vi "Header Footer Transform Header Footer [ ] V3.vi"(7 "Header or Footer [ ]":T15, 11 "error in (no error)":errorcluster) -> (8 "Header or Footer Complete Cluster":T1, 15 "error out":errorcluster)   [LabVIEW 2019, in "Exaprom PDF.lvlib"]
doc: "Version 1.0\nDeveloped by Jean-Marc Simard\nCopyright © 2010, Exaprom Inc.\nAll rights reserved.\nLicense: BSD\n\nWith iTextSharp 4.1.6 (http://itextsharp.sourceforge.net)\nunder Mozilla Public License Version 1.1\n(http://www.mozilla.org/MPL/MPL-1.1.html)"
uses:
  Exaprom PDF.lvlib
  LV Class/Header and Footer Class/VIs/Controls/Header Footer [ ] V2.ctl
  LV Class/Header and Footer Class/VIs/Controls/Header Footer cluster V2.ctl
  Controls/Header, Footer and Watermark Controls/Header or Footer.ctl
  Controls/Header, Footer and Watermark Controls/Header Footer Type.ctl
  Controls/Header, Footer and Watermark Controls/Header footer horiz alignment.ctl
  Controls/Table Controls/Cell Vertical alignment.ctl
  Controls/Text Controls/Line spacing.ctl
  Controls/Header, Footer and Watermark Controls/Page number.ctl
  Controls/Font Controls/Font complete cluster horizontal.ctl
  Controls/Font Controls/Font size.ctl
  Controls/Font Controls/Font color.ctl
  Controls/Font Controls/Type and encoding.ctl
  Controls/Text Controls/Unicode/Type and run direction.ctl
  C:/work/niobrara_lv/labview pdf writer fixing/DLL/itextsharp.dll
  DLL/itextsharp.dll
  Controls/Header, Footer and Watermark Controls/Header Footer Line.ctl
  Controls/Header, Footer and Watermark Controls/Header Footer Complete Cluster.ctl
  Controls/Header, Footer and Watermark Controls/Header or Footer Position.ctl
  Controls/Header, Footer and Watermark Controls/Header Footer Cluster with references.ctl
  Controls/Text Controls/Text type.ctl
  LV Class/Header and Footer Class/Header and Footer Class.lvclass
panel:
  # "X"
  # "Y"
  # "X"
  # "Y"
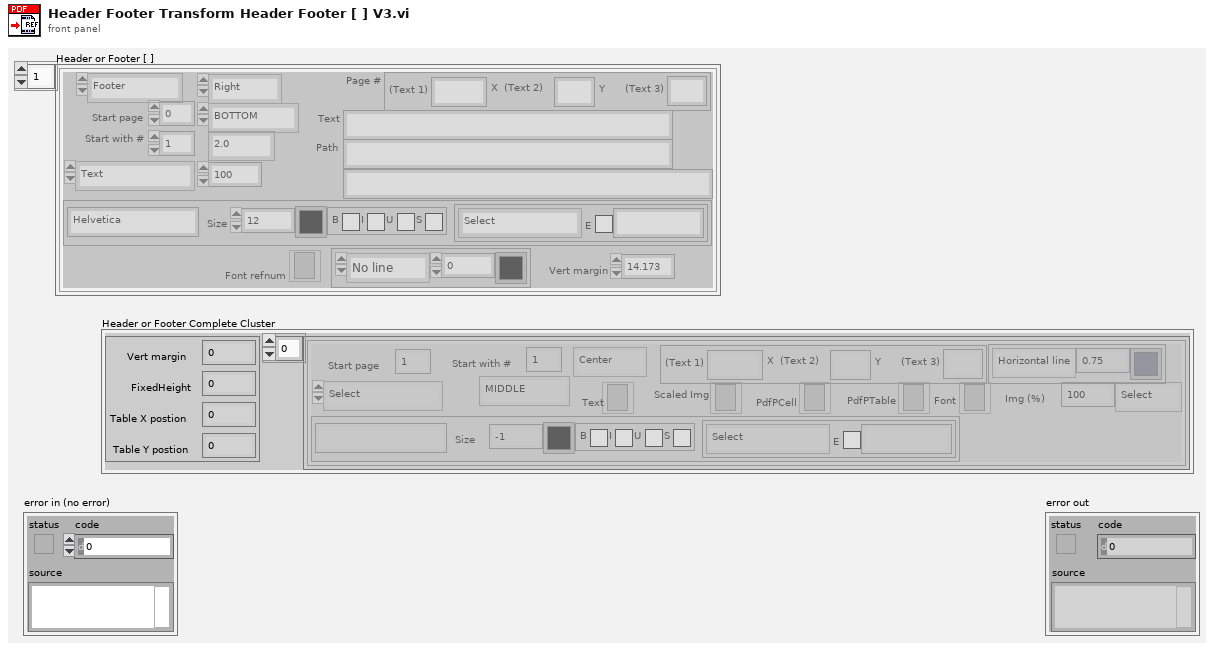
[diagram p1: front panel]
types:
  T1 = typedef "Exaprom PDF.lvlib/Header Footer Complete Cluster.ctl" = cluster{"Table position":T2, "Header Footer Cluster with references [ ]":T3[]}
  T2 = typedef "Exaprom PDF.lvlib/Header or Footer Position.ctl" = cluster{"Vert margin":dbl, "FixedHeight":dbl, "Table X postion":dbl, "Table Y postion":dbl}
  T3 = typedef "Exaprom PDF.lvlib/Header Footer Cluster with references.ctl" = cluster{"Start page":i32, "Type":T4, "Start with #":i32, "Alignment":T5, "Vertical Alignement":T6, "Page #":T7, "Text":refnum<k24>, "Scaled Img":refnum<k24>, "PdfPCell":refnum<k24>, "PdfPTable":refnum<k24>, "Font Cluster":T8, "Font ":refnum<k24>, "Img (%)":sgl, "Line":cluster{"Line":T13, "Thickness (points)":sgl, "Colour":T10}, "Line spacing":T14}
  T4 = typedef "Exaprom PDF.lvlib/Header Footer Type.ctl" = enum16{"Select", "Text", "Text + hyperlink", "Page number", "Image", "Image + hyperlink"}
  T5 = typedef "Exaprom PDF.lvlib/Header footer horiz alignment.ctl" = enum16{"Left", "Center", "Right"}
  T6 = typedef "Exaprom PDF.lvlib/Cell Vertical alignment.ctl" = enum16{"TOP", "MIDDLE", "BOTTOM"}
  T7 = typedef "Exaprom PDF.lvlib/Page number.ctl" = cluster{"Text 1":string, "Text 2":string, "Text 3":string}
  T8 = typedef "Exaprom PDF.lvlib/Font complete cluster horizontal.ctl" = cluster{"Name":string, "Size":T9, "Color":T10, "Style":cluster{"Bold":bool, "Italic":bool, "Underline":bool, "Strikeout":bool}, "Type":T11}
  T9 = typedef "Exaprom PDF.lvlib/Font size.ctl" = sgl
  T10 = typedef "Exaprom PDF.lvlib/Font color.ctl" = u32
  T11 = typedef "Exaprom PDF.lvlib/Type and encoding.ctl" = cluster{"Type&direction":T12, "Embedded":bool, "Encoding":string}
  T12 = typedef "Exaprom PDF.lvlib/Type and run direction.ctl" = enum16{"Select", "ASCII", "UTF-16", "UTF-16 (default)", "UTF-16 (LTR)", "UTF-16 (RTL)"}
  T13 = typedef "Exaprom PDF.lvlib/Header Footer Line.ctl" = enum16{"No line", "Horizontal line"}
  T14 = typedef "Exaprom PDF.lvlib/Line spacing.ctl" = enum16{"Select", "1.0", "1.5", "2.0"}
  T15 = typedef "Exaprom PDF.lvlib/Header and Footer Class.lvclass/Header Footer [ ] V2.ctl" = T16[]
  T16 = typedef "Exaprom PDF.lvlib/Header and Footer Class.lvclass/Header Footer cluster V2.ctl" = cluster{"Header or Footer":T17, "Start page":i32, "Start with #":i32, "Type":T4, "Alignment":T5, "Vertical Alignement":T6, "Line spacing":T14, "Image (%)":sgl, "Page #":T7, "Text":string, "Path":string, "Font":T8, "Font refnum":refnum<k24>, "Line":cluster{"Line":T13, "Thickness (points)":sgl, "Colour":T10}, "Vert margin":dbl, "Hyperlink":string}
  T17 = typedef "Exaprom PDF.lvlib/Header or Footer.ctl" = enum16{"Header", "Footer"}
  T18 = typedef "Exaprom PDF.lvlib/Text type.ctl" = enum16{"empty", "Text", "Hyperlink"}
  T19 = cluster{"Text type":T18, "Text":string, "Hyperlink":string}[]
  T20 = cluster{"Text type":T18, "Text":string, "Hyperlink":string}
  T21 = cluster{"Line":T13, "Thickness (points)":sgl, "Colour":T10}
  T22 = cluster{"Table position":T2, "Header Footer Cluster with references [ ]":T3[]}
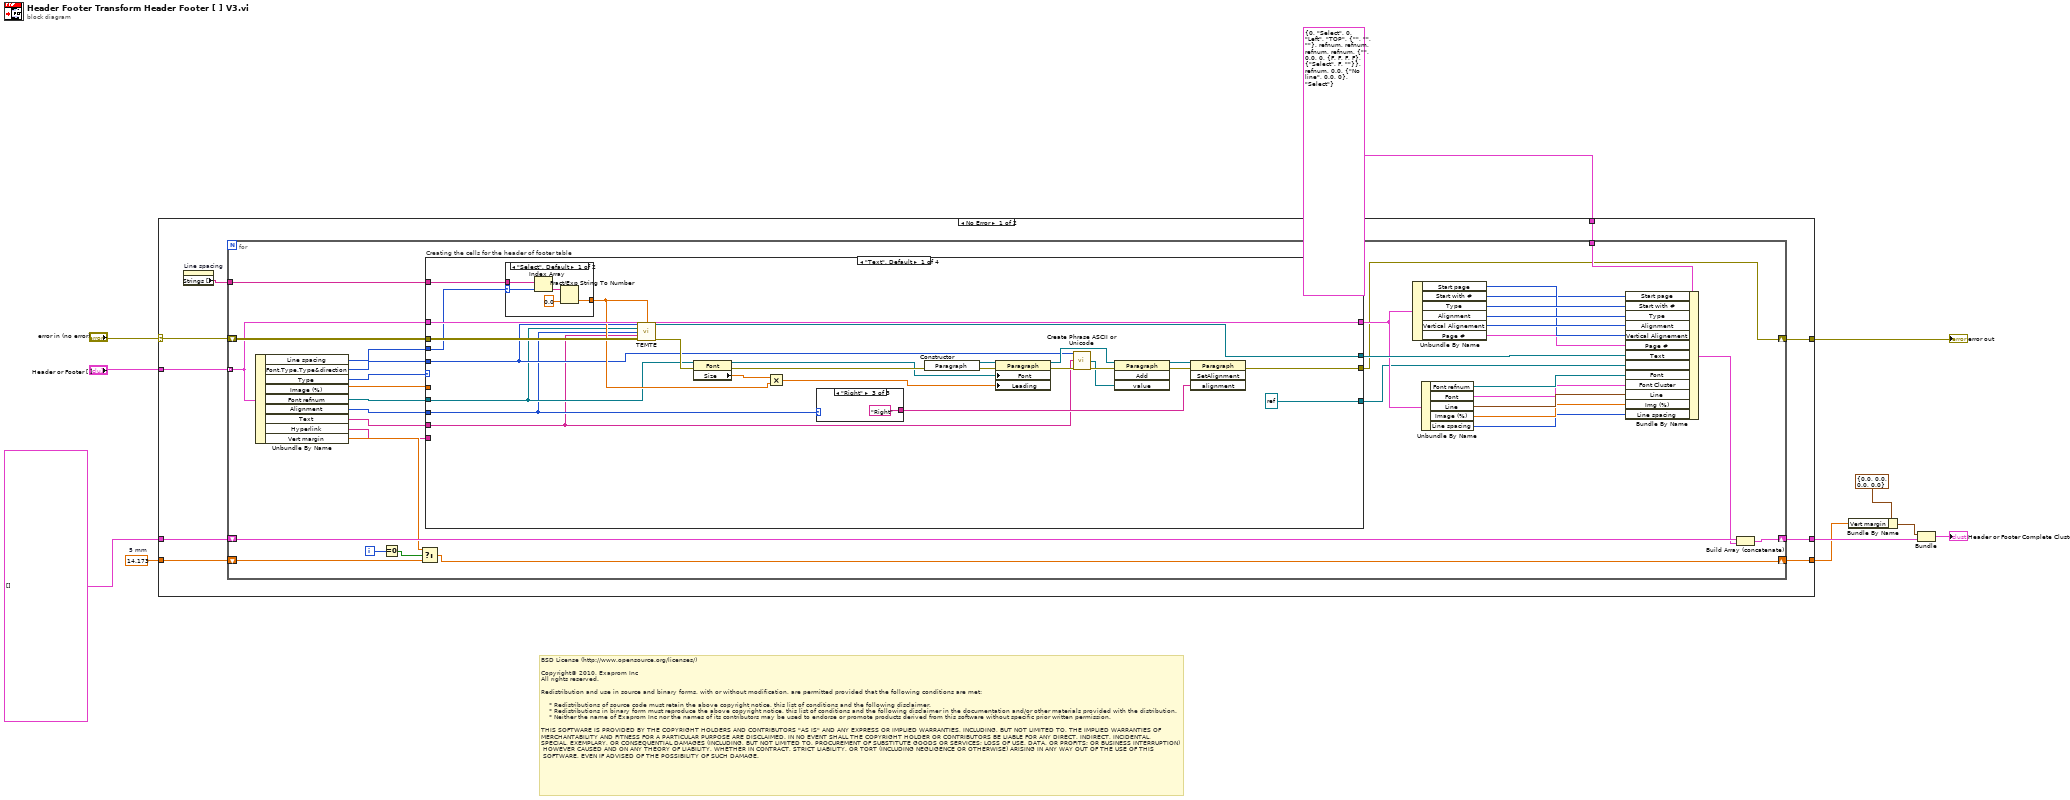
[diagram p0: block diagram]
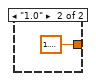
[diagram p2: hidden frame]
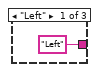
[diagram p3: hidden frame]
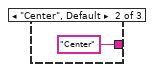
[diagram p4: hidden frame]
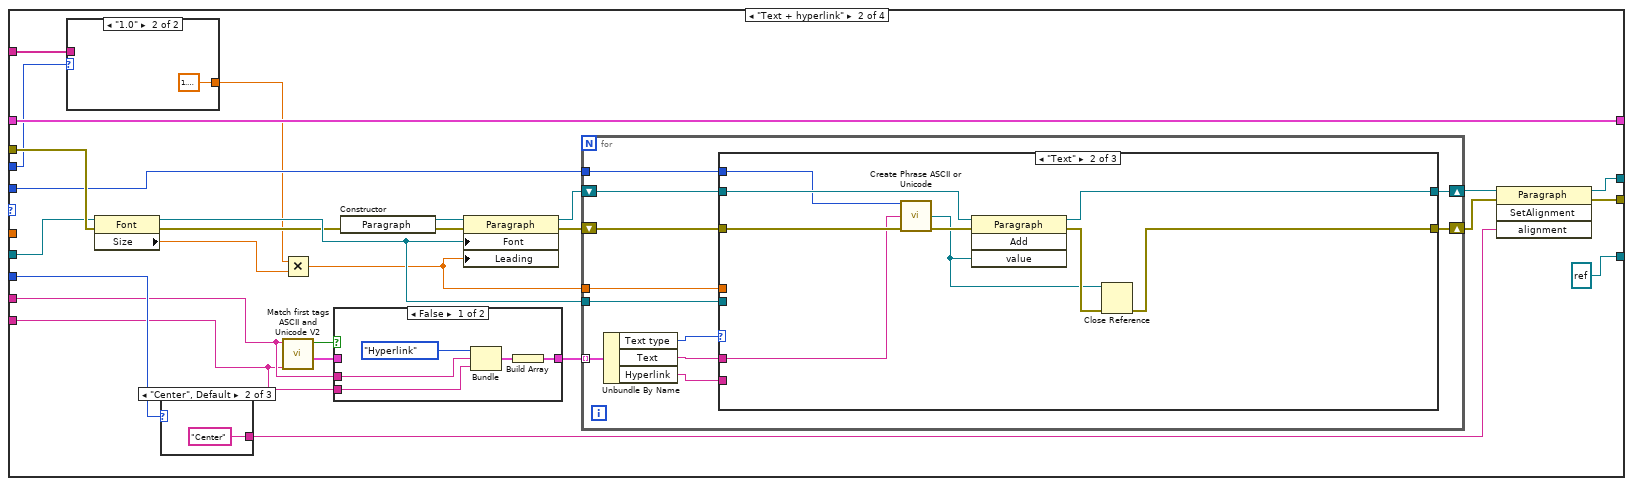
[diagram p5: hidden frame]
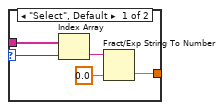
[diagram p6: hidden frame]
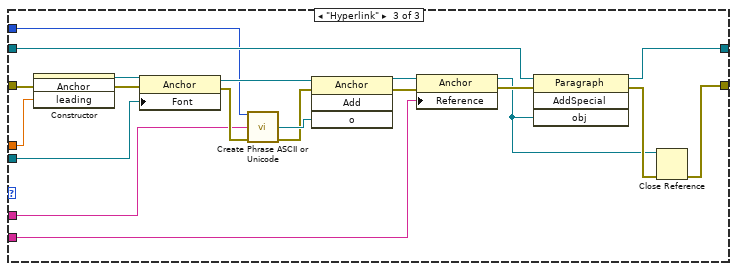
[diagram p9: hidden frame]
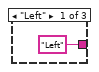
[diagram p10: hidden frame]
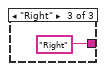
[diagram p11: hidden frame]
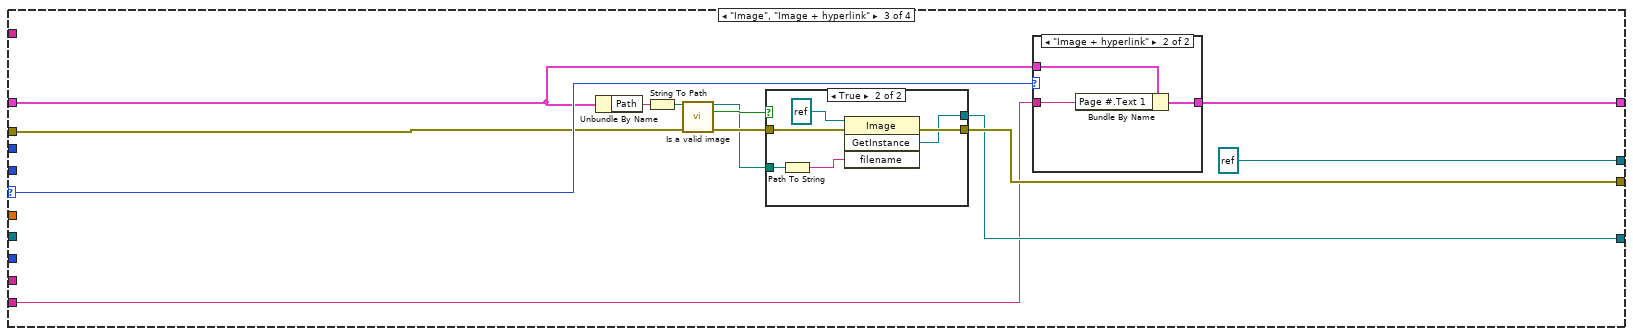
[diagram p12: hidden frame]
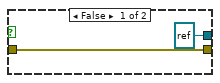
[diagram p13: hidden frame]
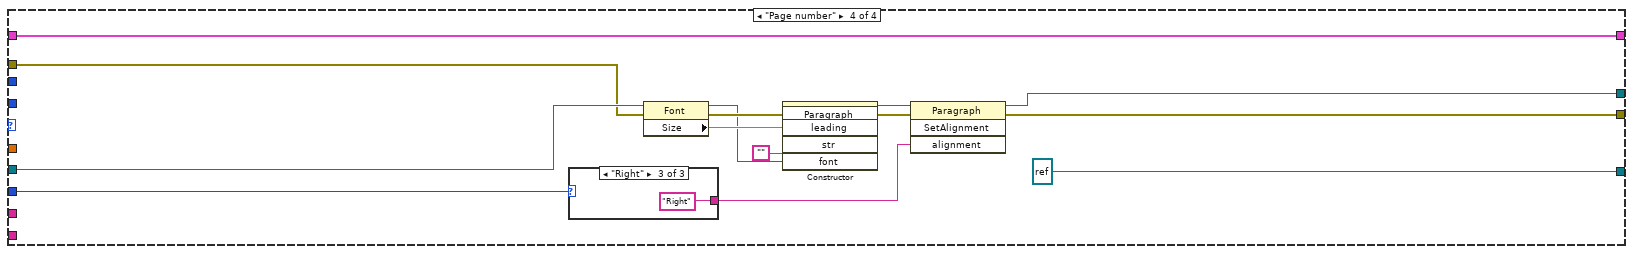
[diagram p15: hidden frame]
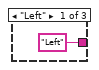
[diagram p16: hidden frame]
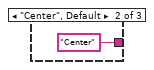
[diagram p17: hidden frame]
diagram:
  w5 = 14.173  # 5 mm
  # "BSD License (http://www.opensource.org/licenses/)\n\nCopyright© 2010, Exaprom Inc\nAll rights reserved.\n\nRedistribution and use in source and binary forms, with or without modification, are permitted provided that the following conditions are met:\n\n    * Redistributions of source code must retain the above copyright notice, this list of conditions and the following disclaimer.\n    * Redistributions in binary form must reproduce the above copyright notice, this list of conditions and the following disclaimer in the documentation and/or other materials provided with the distribution.\n    * Neither the name of Exaprom Inc nor the names of its contributors may be used to endorse or promote products derived from this software without specific prior written permission.\n\nTHIS SOFTWARE IS PROVIDED BY THE COPYRIGHT HOLDERS AND CONTRIBUTORS \"AS IS\" AND ANY EXPRESS OR IMPLIED WARRANTIES, INCLUDING, BUT NOT LIMITED TO, THE IMPLIED WARRANTIES OF \nMERCHANTABILITY AND FITNESS FOR A PARTICULAR PURPOSE ARE DISCLAIMED. IN NO EVENT SHALL THE COPYRIGHT HOLDER OR CONTRIBUTORS BE LIABLE FOR ANY DIRECT, INDIRECT, INCIDENTAL,\nSPECIAL, EXEMPLARY, OR CONSEQUENTIAL DAMAGES (INCLUDING, BUT NOT LIMITED TO, PROCUREMENT OF SUBSTITUTE GOODS OR SERVICES; LOSS OF USE, DATA, OR PROFITS; OR BUSINESS INTERRUPTION)\n HOWEVER CAUSED AND ON ANY THEORY OF LIABILITY, WHETHER IN CONTRACT, STRICT LIABILITY, OR TORT (INCLUDING NEGLIGENCE OR OTHERWISE) ARISING IN ANY WAY OUT OF THE USE OF THIS\n SOFTWARE, EVEN IF ADVISED OF THE POSSIBILITY OF SUCH DAMAGE."
  n1 = case shown="No Error" "error in (no error)" {
    selector: "error in (no error)" -> [w16 w219]
    tunnel: "Header or Footer [ ]" -> [w15 _]
    tunnel: [w20 w219] -> w11
    tunnel: T3 {"Start page"=0, "Type"=enum."Select", "Start with #"=0, "Alignment"=enum."Left", "Vertical Alignement"=enum."TOP", "Page #"={"Text 1"="", "Text 2"="", "Text 3"=""}, "Text"=refnum, "Scaled Img"=refnum, "PdfPCell"=refnum, "PdfPTable"=refnum, "Font Cluster"={"Name"="", "Size"=0.0, "Color"=0, "Style"={"Bold"=FALSE, "Italic"=FALSE, "Underline"=FALSE, "Strikeout"=FALSE}, "Type"={"Type&direction"=enum."Select", "Embedded"=FALSE, "Encoding"=""}}, "Font "=refnum, "Img (%)"=0.0, "Line"={"Line"=enum."No line", "Thickness (points)"=0.0, "Colour"=0}, "Line spacing"=enum."Select"} ("Header Footer Cluster with references") -> [w19 _]
    tunnel: T3[] [] ("Header Footer Cluster with references [ ]") -> [w18 w218]
    tunnel: [w17 w218] -> w7
    tunnel: [w14 w217] -> w2
    tunnel: w5 -> [w13 w217]
    frame No Error {
      n2 = property on="Line spacing" class="Enum (strict)"() -> ("Strings []"=w12:string[])  [unwired: 2 in, 2 out]
      n3 = for {
        tunnel: w15 -> [w41] mode=indexing
        tunnel: w19 -> [w50]
        shift-right: [w43] -> w17
        shift-left: w18 -> [w42]
        shift-right: [w36] -> w20
        shift-left: w16 -> [w39]
        shift-right: [w29] -> w14
        shift-left: w13 -> [w30]
        tunnel: w12 -> [w22]
        i -> [w32]
        n4 = Unbundle By Name(w41) -> ("Line spacing"=w23:T14, "Font.Type.Type&direction"=w27:T12, "Type"=w52:T4, "Image (%)"=w53:sgl, "Font refnum"=w55:refnum<k24>, "Alignment"=w54:T5, "Text"=w51:string, "Hyperlink"=w25:string, "Vert margin"=w26:dbl)
        n5 = Equal To 0?(x=w32) -> (x = 0?=w31:bool)
        n6 = Select(t=w26, s=w31, f=w30) -> (s? t:f=w29:dbl)
        n7 = case "Creating the cells for the header of footer table" shown="\"Text\", Default" w52 {
          selector: w52 -> [_ _ w185 _]
          tunnel: w41 -> [w78 w114 w180 w208]
          tunnel: w55 -> [w59 w99 _ w213]
          tunnel: w54 -> [w58 w117 _ w212]
          tunnel: w53 -> [_ _ _ _]
          tunnel: w51 -> [w57 w102 _ _]
          tunnel: w39 -> [w81 w100 w177 w211]
          tunnel: [w56 w112 refnum<k24> refnum ("new reference") w207] -> w44
          tunnel: [refnum<k24> refnum ("GetInstanceImage OUT") refnum<k24> refnum ("GetInstanceImage OUT") w183 refnum<k24> refnum ("GetInstanceImage OUT")] -> w38
          tunnel: [w80 w115 w186 w210] -> w36
          tunnel: [w78 w114 w184 w208] -> w40
          tunnel: w27 -> [w60 w98 _ _]
          tunnel: w25 -> [_ w101 w175 _]
          tunnel: w23 -> [w63 w92 _ _]
          tunnel: w22 -> [w65 w93 _ _]
          frame "Text", Default {
            n8 = case shown="\"Select\", Default" w63 {
              selector: w63 -> [w82 _]
              tunnel: w65 -> [w84 _]
              tunnel: [w83 sgl 1.1] -> w61
              frame "Select", Default {
                n9 = Index Array(array=w84, index=w82) -> (element=w86:string)
                n10 = Fract/Exp String To Number(string=w86, default (0 dbl)=sgl 0.0 ("default (0 DBL)")) -> (number=w83:sgl)  [unwired: 3 out]
              }
              frame "1.0" {
              }
            }
            n11 = call "TEMTE.vi"("Type and run direction"=w60, "LS Multiplier"=w61, "Font refnum"=w59, "Alignment"=w58, "Text"=w57, "error in (no error)"=w81) -> ("Paragraph"=w56:refnum<k24>, "error out"=w62:errorcluster)  [unwired: 8 in]
            n12 = property class="Font"(reference=w59, error in=w62) -> (reference out=w73:refnum<k24>, error out=w76:errorcluster, "Size"=w72:sgl)
            n13 = Multiply(x=w72, y=w61) -> (x*y=w64:sgl)
            n14 = case shown="\"Right\"" w58 {
              tunnel: ["Left" "Center" "Right"] -> w77
              frame "Left" {
              }
              frame "Center", Default {
              }
              frame "Right" {
              }
            }
            n15 = constructor class="Paragraph"(error in=w76) -> (reference out=w74:refnum<k24>, error out=w75:errorcluster)  [unwired: 2 in, 1 out]
            n16 = property class="Paragraph"(reference=w74, error in=w75, "Font"=w73, "Leading"=w64) -> (reference out=w69:refnum<k24>, error out=w68:errorcluster)
            n17 = call "Create Phrase ASCII or Unicode.vi"("Character type"=w60, "Text"=w57, "error in (no error)"=w68) -> ("Phrase refnum"=w66:refnum<k24>, "error out"=w67:errorcluster)  [unwired: 10 in, 1 out]
            n18 = invoke class="Paragraph" method="Add"(reference=w69, error in=w67, "value"=w66) -> (reference out=w71:refnum<k24>, error out=w70:errorcluster)  [unwired: 1 in, 2 out]
            n19 = invoke class="Paragraph" method="SetAlignment"(reference=w71, error in=w70, "alignment"=w77) -> (error out=w80:errorcluster)  [unwired: 1 in, 3 out]
          }
          frame "Text + hyperlink" {
            n20 = case shown="\"1.0\"" w92 {
              selector: w92 -> [w118 _]
              tunnel: w93 -> [w120 _]
              tunnel: [w119 sgl 1.1] -> w91
              frame "Select", Default {
                n21 = Index Array(array=w120, index=w118) -> (element=w122:string)
                n22 = Fract/Exp String To Number(string=w122, default (0 dbl)=sgl 0.0 ("default (0 DBL)")) -> (number=w119:sgl)  [unwired: 3 out]
              }
              frame "1.0" {
              }
            }
            n23 = property class="Font"(reference=w99, error in=w100) -> (reference out=w111:refnum<k24>, error out=w106:errorcluster, "Size"=w110:sgl)
            n24 = case shown="\"Center\", Default" w117 {
              tunnel: ["Left" "Center" "Right"] -> w113
              frame "Left" {
              }
              frame "Center", Default {
              }
              frame "Right" {
              }
            }
            n25 = Multiply(x=w91, y=w110) -> (x*y=w94:sgl)
            n26 = call "Match first tags ASCII and Unicode V2.vi"("Hyperlink"=w101, "Text"=w102) -> ("Array"=w109:T19, "Find tag ?"=w107:bool)  [unwired: 3 in, 5 out]
            n27 = case shown="False" w107 {
              tunnel: [w124 w129] -> w108
              tunnel: w109 -> [_ w129]
              tunnel: w102 -> [w126 _]
              tunnel: w101 -> [w127 _]
              frame False {
                n28 = Bundle("Text type"=Text_type."Hyperlink", "Text"=w126, "Hyperlink"=w127) -> (w128:T20)  [unwired: 1 in]
                n29 = Build Array(w128) -> (w124:T19)
              }
              frame True {
              }
            }
            n30 = constructor class="Paragraph"(error in=w106) -> (reference out=w104:refnum<k24>, error out=w105:errorcluster)  [unwired: 2 in, 1 out]
            n31 = property class="Paragraph"(reference=w104, error in=w105, "Font"=w111, "Leading"=w94) -> (reference out=w95:refnum<k24>, error out=w103:errorcluster)
            n32 = for {
              shift-right: [w138] -> w96
              shift-left: w95 -> [w139]
              shift-right: [w137] -> w97
              shift-left: w103 -> [w140]
              tunnel: w108 -> [w136] mode=indexing
              tunnel: w94 -> [w132]
              tunnel: w111 -> [w131]
              tunnel: w98 -> [w130]
              n33 = Unbundle By Name(w136) -> ("Text type"=w135:T18, "Text"=w134:string, "Hyperlink"=w133:string)
              n34 = case shown="\"Text\"" w135 {
                tunnel: w140 -> [w142 w150 w165]
                tunnel: w139 -> [w141 w149 w160]
                tunnel: [w141 w148 w161] -> w138
                tunnel: [w142 w145 w156] -> w137
                tunnel: w134 -> [_ w147 w159]
                tunnel: w133 -> [_ _ w158]
                tunnel: w132 -> [_ _ w154]
                tunnel: w131 -> [_ _ w153]
                tunnel: w130 -> [_ w143 w152]
                frame "empty", Default {
                }
                frame "Text" {
                  n35 = call "Create Phrase ASCII or Unicode.vi"("Character type"=w143, "Text"=w147, "error in (no error)"=w150) -> ("Phrase refnum"=w144:refnum<k24>, "error out"=w151:errorcluster)  [unwired: 10 in, 1 out]
                  n36 = invoke class="Paragraph" method="Add"(reference=w149, error in=w151, "value"=w144) -> (reference out=w148:refnum<k24>, error out=w146:errorcluster)  [unwired: 1 in, 2 out]
                  n37 = Close Reference(reference=w144, error in (no error)=w146) -> (error out=w145:errorcluster)
                }
                frame "Hyperlink" {
                  n38 = constructor class="Anchor"(error in=w165, "leading"=w154) -> (reference out=w171:refnum<k24>, error out=w170:errorcluster)  [unwired: 2 in, 2 out]
                  n39 = property class="Anchor"(reference=w171, error in=w170, "Font"=w153) -> (reference out=w169:refnum<k24>, error out=w164:errorcluster)
                  n40 = call "Create Phrase ASCII or Unicode.vi"("Character type"=w152, "Text"=w159, "error in (no error)"=w164) -> ("Phrase refnum"=w166:refnum<k24>, "error out"=w163:errorcluster)  [unwired: 10 in, 1 out]
                  n41 = invoke class="Anchor" method="Add"(reference=w169, error in=w163, "o"=w166) -> (reference out=w167:refnum<k24>, error out=w168:errorcluster)  [unwired: 1 in, 2 out]
                  n42 = property class="Anchor"(reference=w167, error in=w168, "Reference"=w158) -> (reference out=w155:refnum<k24>, error out=w162:errorcluster)
                  n43 = invoke class="Paragraph" method="AddSpecial"(reference=w160, error in=w162, "obj"=w155) -> (reference out=w161:refnum<k24>, error out=w157:errorcluster)  [unwired: 1 in, 2 out]
                  n44 = Close Reference(reference=w155, error in (no error)=w157) -> (error out=w156:errorcluster)
                }
              }
            }
            n45 = invoke class="Paragraph" method="SetAlignment"(reference=w96, error in=w97, "alignment"=w113) -> (reference out=w112:refnum<k24>, error out=w115:errorcluster)  [unwired: 1 in, 2 out]
          }
          frame "Image", "Image + hyperlink" {
            n46 = Unbundle By Name(w180) -> ("Path"=w181:string)
            n47 = String To Path(string=w181) -> (path=w182:path)
            n48 = call "Is a valid image.vi"("Image path"=w182, "error in (no error)"=w177) -> ("dup path"=w176:path, "Valid Image?"=w179:bool, "error out"=w178:errorcluster)  [unwired: 11 out]
            n49 = case shown="True" w179 {
              tunnel: w176 -> [_ w194]
              tunnel: [w189 w193] -> w186
              tunnel: [refnum<k24> refnum ("GetInstance") w192] -> w183
              tunnel: w178 -> [w189 w191]
              frame False {
              }
              frame True {
                n50 = Path To String(path=w194) -> (string=w190:string)
                n51 = invoke class="Image" method="GetInstance"(reference=refnum<k24> refnum ("image"), error in=w191, "filename"=w190) -> (error out=w193:errorcluster, "GetInstance"=w192:refnum<k24>)  [unwired: 1 in, 2 out]
              }
            }
            n52 = case shown="\"Image + hyperlink\"" w185 {
              tunnel: [w196 w198] -> w184
              tunnel: w180 -> [w196 w199]
              tunnel: w175 -> [_ w197]
              frame "Select", Default {
              }
              frame "Image + hyperlink" {
                n53 = Bundle By Name(cluster=w199, "Page #.Text 1"=w197) -> (w198:T16)
              }
            }
          }
          frame "Page number" {
            n54 = case shown="\"Right\"" w212 {
              tunnel: ["Left" "Center" "Right"] -> w204
              frame "Left" {
              }
              frame "Center", Default {
              }
              frame "Right" {
              }
            }
            n55 = property class="Font"(reference=w213, error in=w211) -> (reference out=w201:refnum<k24>, error out=w203:errorcluster, "Size"=w202:sgl)
            n56 = constructor class="Paragraph"(error in=w203, "leading"=w202, "str"="", "font"=w201) -> (reference out=w205:refnum<k24>, error out=w200:errorcluster)  [unwired: 2 in, 4 out]
            n57 = invoke class="Paragraph" method="SetAlignment"(reference=w205, error in=w200, "alignment"=w204) -> (reference out=w207:refnum<k24>, error out=w210:errorcluster)  [unwired: 1 in, 2 out]
          }
        }
        n58 = Unbundle By Name(w40) -> ("Start page"=w28:i32, "Start with #"=w49:i32, "Type"=w48:T4, "Alignment"=w47:T5, "Vertical Alignement"=w46:T6, "Page #"=w45:T7)
        n59 = Unbundle By Name(w40) -> ("Font refnum"=w34:refnum<k24>, "Font"=w21:T8, "Line"=w35:T21, "Image (%)"=w33:sgl, "Line spacing"=w24:T14)
        n60 = Bundle By Name(cluster=w50, "Start page"=w28, "Start with #"=w49, "Type"=w48, "Alignment"=w47, "Vertical Alignement"=w46, "Page #"=w45, "Text"=w44, "Scaled Img"=w38, "Font"=w34, "Font Cluster"=w21, "Line"=w35, "Img (%)"=w33, "Line spacing"=w24) -> (w37:T3)
        n61 = Build Array (concatenate)(w42, w37) -> (w43:T3[])
      }
    }
    frame Error {
    }
  }
  "error out" <- w11
  n62 = Bundle By Name(cluster=T2 {"Vert margin"=0.0, "FixedHeight"=0.0, "Table X postion"=0.0, "Table Y postion"=0.0} ("Table position"), "Vert margin"=w2) -> (w3:T2)
  n63 = Bundle("Table position"=w3, "Header Footer Cluster with references [ ]"=w7) -> (→"Header or Footer Complete Cluster":T22)  [unwired: 1 out]
